vi "MPM_Set_Logging_Data_Point.vi"(8 "error in (no error)":errorcluster, 10 "count":i32, 11 ".NET Reference in":refnum<k24>) -> (0 "error out":errorcluster, 3 "Reference out":refnum<k24>)   [LabVIEW 2017]
uses:
  D:/test/FULLband-sts/Fullband_Sample/DLL/InstrumentDLL.dll
  DLL/InstrumentDLL.dll
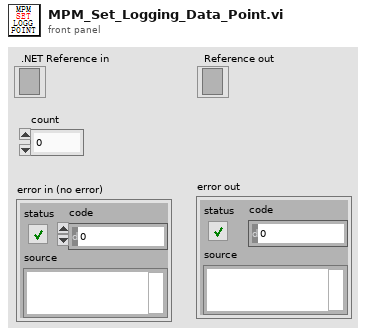
[diagram p1: front panel]
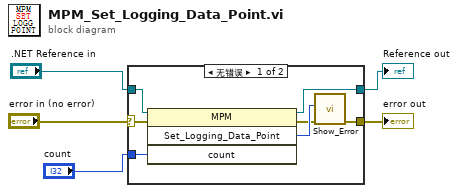
[diagram p0: block diagram]
diagram:
  n1 = case shown="无错误" "error in (no error)" {
    selector: "error in (no error)" -> [w6 w14]
    tunnel: ".NET Reference in" -> [w12 w13]
    tunnel: [w11 w13] -> w4
    tunnel: "count" -> [w10 _]
    tunnel: [w7 w14] -> w2
    frame No Error {
      n2 = invoke class="MPM" method="Set_Logging_Data_Point"(reference=w12, error in=w6, "count"=w10) -> (reference out=w11:refnum<k24>, error out=w8:errorcluster, "Set_Logging_Data_Point"=w9:i32)  [unwired: 1 in, 1 out]
      n3 = call "Show_Error.vi"("error in (no error)"=w8, "Error"=w9) -> ("error out"=w7:errorcluster)  [unwired: 9 in]
    }
    frame Error {
    }
  }
  "Reference out" <- w4
  "error out" <- w2
